vi "Monitor_grey.vi"() -> ()   [LabVIEW 2016]
uses:
  <vilib>/Utility/file.llb/Write Delimited Spreadsheet (string).vi
  <vilib>/MakerHub/Toolbox/LMH-Toolbox.lvlib
panel:
  in  "Tab Control":enum32{"Page 1", "Page 2"}(tab)=enum."Page 2"
  out "2 Terminal Conductance":cluster{"Y":dbl[], "Y":dbl[]}[](graph)
  out "4 Terminal Resistance":cluster{"Y":dbl[], "Y":dbl[]}[](graph)
  in  "Stop":bool
  in  "Comments":string="Test"
  in  "base path":path=path "C:/Users/ansom/Desktop/Monitor/20180205"
  in  "folder name":string="monitor cond"
  in  "filename":string="Test"
  in  "Reset":bool
  in  "Excitation voltage":dbl=0.1
  in  "Diff Voltage?":bool
  in  "Current (I-)":i32
  in  "Voltage Pairs (+, -,...)":i32[][](array[numeric])=[[0, 1, 1, 2], [2, 3, 4, 3]]
  in  "wait (ms)":u32=60
  out "Temperature":dbl=27.13
  out "Humidity":dbl=35.08
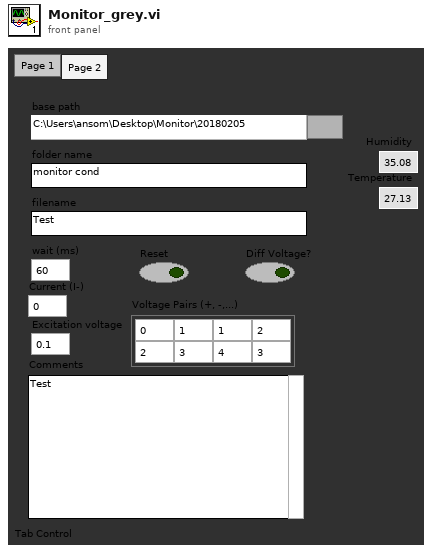
[diagram p1: front panel]
types:
  T1 = typedef "LVPositionTypeDef.ctl" = cluster{"Left":i32, "Top":i32}
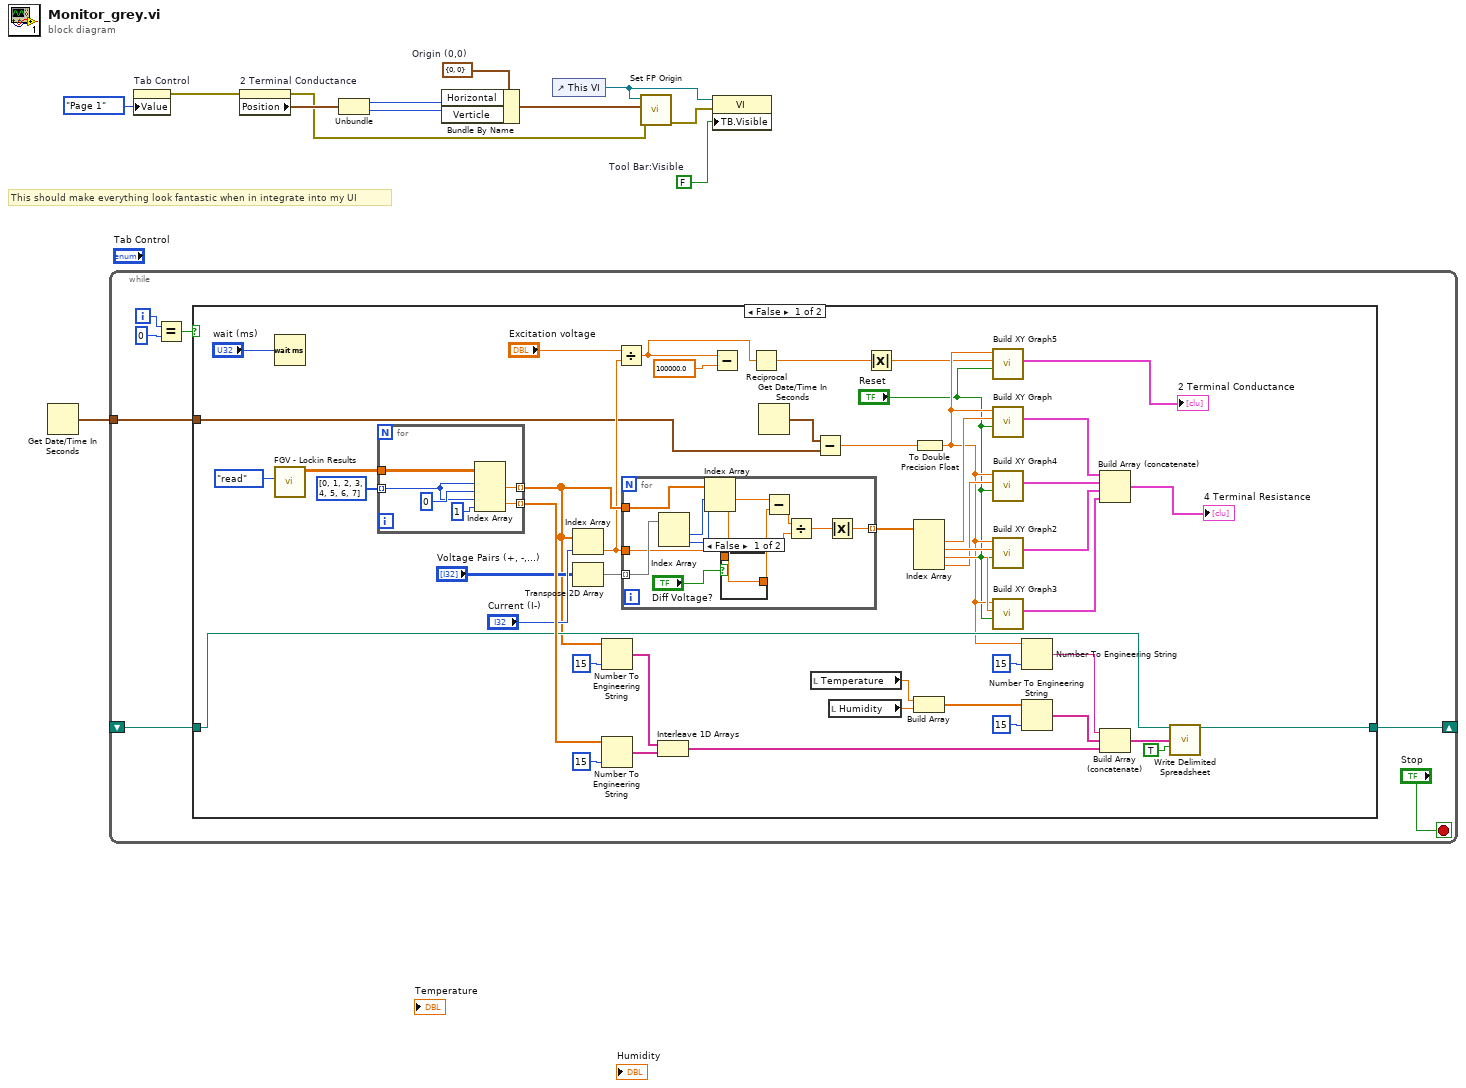
[diagram p0: block diagram]
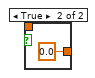
[diagram p2: hidden frame]
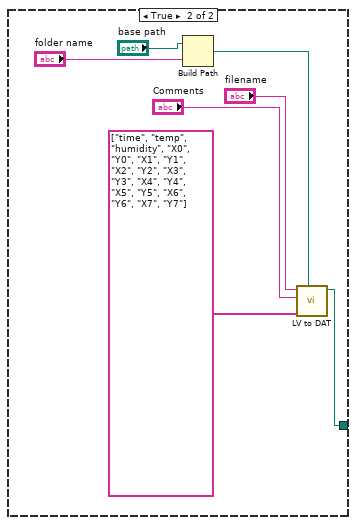
[diagram p3: hidden frame]
diagram:
  w5 = FALSE  # Tool Bar:Visible
  w12 = cluster{"Horizontal":i16, "Verticle":i16} {"Horizontal"=0, "Verticle"=0}  # Origin (0,0)
  # "This should make everything look fantastic when in integrate into my UI"
  n1 = Get Date/Time In Seconds() -> (seconds since 1Jan1904=w4:timestamp)
  n2 = while {
    shift-right: [w16] -> _
    shift-left: _ -> [w15]
    tunnel: w4 -> [w14]
    i -> [w19]
    stop <- "Stop" stop-if-true
    n3 = Equal?(x=w19, y=0) -> (x = y?=w17:bool)
    n4 = case shown="False" w17 {
      tunnel: [w54 w87] -> w16
      tunnel: w15 -> [w57 _]
      tunnel: w14 -> [w27 _]
      frame False {
        n5 = Wait (ms)(milliseconds to wait="wait (ms)") -> ()  [unwired: 1 out]
        n6 = call <userlib>:"FGV - Lockin Results.vi"("Function"=enum16{"write", "read"}."read") -> ("Results"=w64:dbl[][])  [unwired: 5 in, 1 out]
        n7 = for {
          tunnel: w64 -> [w83]
          tunnel: i32[] [0, 1, 2, 3, 4, 5, 6, 7] ("Lockins") -> [w84] mode=indexing
          tunnel: [w81] -> w42 mode=indexing
          tunnel: [w82] -> w58 mode=indexing
          n8 = Index Array(array=w83, index (row) #1=w84, index (col) #1=0 ("disabled index (col)"), index (row) #2=w84, index (col) #2=1 ("disabled index (col)")) -> (element #1=w81:dbl, element #2=w82:dbl)
        }
        n9 = Index Array(array=w42, index="Current (I-)") -> (element=w29:dbl)
        n10 = Transpose 2D Array(2D array="Voltage Pairs (+, -,...)") -> (transposed array=w43:i32[][])
        n11 = Number To Engineering String(2:i16 15 ("precision (6)"), 4:w42) -> (0:w61:string[])  [unwired: 2 out]
        n12 = Number To Engineering String(2:i16 15 ("precision (6)"), 4:w58) -> (0:w60:string[])  [unwired: 2 out]
        n13 = Divide(x="Excitation voltage", y=w29) -> (x/y=w24:dbl)
        n14 = for {
          tunnel: w43 -> [w78] mode=indexing
          tunnel: w42 -> [w77]
          tunnel: w29 -> [w73]
          tunnel: [w70] -> w41 mode=indexing
          n15 = Index Array(array=w78) -> (element #1=w76:i32, element #2=w75:i32)  [unwired: 2 in]
          n16 = Index Array(array=w77, index #1=w76, index #2=w75) -> (element #1=w74:dbl, element #2=w67:dbl)
          n17 = case shown="False" "Diff Voltage?" {
            tunnel: [w79 0.0] -> w68
            tunnel: w67 -> [w79 _]
            frame False {
            }
            frame True {
            }
          }
          n18 = Subtract(x=w74, y=w68) -> (x-y=w72:dbl)
          n19 = Divide(x=w72, y=w73) -> (x/y=w71:dbl)
          n20 = Absolute Value(x=w71) -> (abs(x)=w70:dbl)
        }
        n21 = Interleave 1D Arrays(w61, w60) -> (w59:string[])
        n22 = Subtract(x=w24, y=100000.0) -> ()  [unwired: 1 out]
        n23 = Reciprocal(x=w24) -> (1/x=w23:dbl)
        n24 = Get Date/Time In Seconds() -> (seconds since 1Jan1904=w28:timestamp)
        n25 = local read "Temperature"() -> (w53:dbl)
        n26 = Subtract(x=w28, y=w27) -> (x-y=w26:dbl)
        n27 = local read "Humidity"() -> (w52:dbl)
        n28 = Absolute Value(x=w23) -> (abs(x)=w22:dbl)
        n29 = Index Array(array=w41) -> (element #1=w40:dbl, element #2=w39:dbl, element #3=w38:dbl, element #4=w37:dbl)  [unwired: 4 in]
        n30 = Build Array(w53, w52) -> (w47:dbl[])
        n31 = To Double Precision Float(number=w26) -> (double precision float=w32:dbl)
        n32 = call "Build XY Graph5"("Reset"="Reset", "Y Input"=w22, "X Input"=w32) -> ("XY Graph"=→"2 Terminal Conductance":cluster{"Y":dbl[], "Y":dbl[]}[])  [unwired: 2 in, 6 out]
        n33 = call "Build XY Graph"("Reset"="Reset", "Y Input"=w40, "X Input"=w32) -> ("XY Graph"=w36:cluster{"Y":dbl[], "Y":dbl[]}[])  [unwired: 2 in, 6 out]
        n34 = call "Build XY Graph4"("Reset"="Reset", "Y Input"=w37, "X Input"=w32) -> ("XY Graph"=w35:cluster{"Y":dbl[], "Y":dbl[]}[])  [unwired: 2 in, 6 out]
        n35 = call "Build XY Graph2"("Reset"="Reset", "Y Input"=w39, "X Input"=w32) -> ("XY Graph"=w34:cluster{"Y":dbl[], "Y":dbl[]}[])  [unwired: 2 in, 6 out]
        n36 = call "Build XY Graph3"("Reset"="Reset", "Y Input"=w38, "X Input"=w32) -> ("XY Graph"=w33:cluster{"Y":dbl[], "Y":dbl[]}[])  [unwired: 2 in, 6 out]
        n37 = Number To Engineering String(2:i16 15 ("precision (6)"), 4:w32) -> (0:w49:string)  [unwired: 2 out]
        n38 = Number To Engineering String(2:i16 15 ("precision (6)"), 4:w47) -> (0:w46:string[])  [unwired: 2 out]
        n39 = Build Array (concatenate)(w36, w35, w34, w33) -> (→"4 Terminal Resistance":cluster{"Y":dbl[], "Y":dbl[]}[])
        n40 = Build Array (concatenate)(w49, w46, w59) -> (w55:string[])
        n41 = call-poly <vilib>:"Write Delimited Spreadsheet.vi"("file path (dialog if empty)"=w57, "1D data"=w55, "append to file? (new file:F)"=TRUE) -> ("new file path (Not A Path if cancelled)"=w54:path)  [unwired: 11 in, 1 out]
      }
      frame True {
        n42 = Build Path(base path="base path", name or relative path="folder name") -> (appended path=w89:path)
        n43 = call <userlib>:"LV to DAT.vi"("path"=w89, "wavenames (.Vx, etc)"=string[] ["time", "temp", "humidity", "X0", "Y0", "X1", "Y1", "X2", "Y2", "X3", "Y3", "X4", "Y4", "X5", "Y5", "X6", "Y6", "X7", "Y7"], "Comments"="Comments", "filename"="filename") -> ("new file path (Not A Path if cancelled)"=w87:path)  [unwired: 7 in]
      }
    }
  }
  n44 = property on="Tab Control" class="TabCtl (strict)"("Value"=enum32{"Page 1", "Page 2"}."Page 1" ("Tab Control")) -> (error out=w2:errorcluster)  [unwired: 2 in, 1 out]
  n45 = property on="2 Terminal Conductance" class="XYGraph (strict)"(error in=w2) -> (error out=w1:errorcluster, "Position"=w11:T1)  [unwired: 1 in, 1 out]
  n46 = Unbundle(w11) -> ("Left"=w10:i32, "Top"=w9:i32)
  n47 = Bundle By Name(cluster=w12, "Horizontal"=w10, "Verticle"=w9) -> (w8:cluster{"Horizontal":i16, "Verticle":i16})
  n48 = control-ref of="This VI"() -> (w7:refnum<vi>)
  n49 = call <vilib>:"Set FP Origin.vi"("Error In"=w1, "Origin (0,0)"=w8, "VI Ref"=w7) -> ("Error Out"=w6:errorcluster)  [unwired: 8 in]
  n50 = property class="VI"(reference=w7, error in=w6, "TB.Visible"=w5) -> ()  [unwired: 2 out]
